vi "initialize_reactors.vi"(8 "ERROR IN":errorcluster, 11 "REACTORS TO USE":u32[](array[numeric])) -> (0 "ERROR OUT":errorcluster, 3 "REACTORS":T1)   [LabVIEW 2013]
uses:
  type_defs/reactors.ctl
  type_defs/reactor.ctl
panel:
  in  "SUMMARY STAT":dbl[](array[numeric])
  in  "TIME STAMPS":dbl[](array[numeric])
  in  "LAST MEASUREMENT":dbl[][](array[numeric])
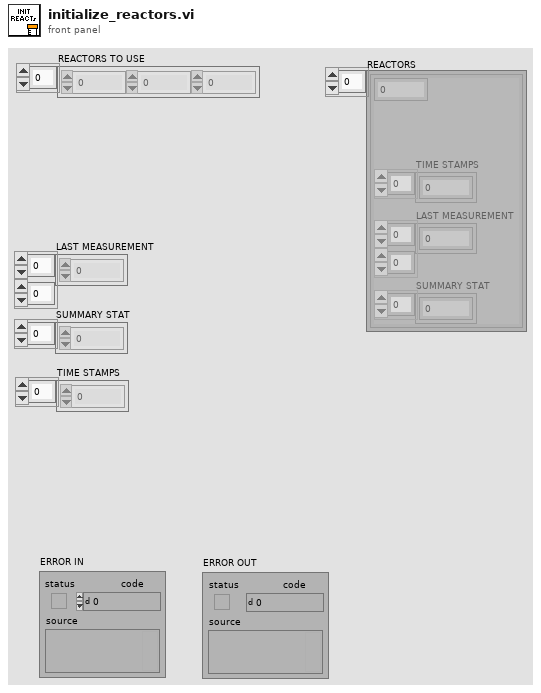
[diagram p1: front panel]
types:
  T1 = typedef "reactors.ctl" = cluster{i32, "TIME STAMPS":dbl[], "LAST MEASUREMENT":T2[][], "SUMMARY STAT":dbl[]}[]
  T2 = typedef "reactor.ctl" = dbl
  T3 = cluster{"Numeric":u32, "TIME STAMPS":dbl[], "LAST MEASUREMENT":dbl[][], "SUMMARY STAT":dbl[]}
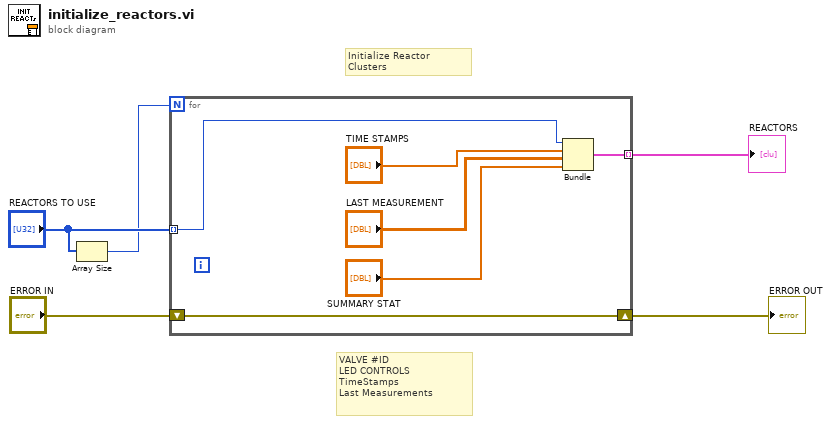
[diagram p0: block diagram]
diagram:
  # "VALVE #ID \nLED CONTROLS\nTimeStamps\nLast Measurements"
  # "Initialize Reactor Clusters"
  n1 = Array Size(array="REACTORS TO USE") -> (size(s)=w2:i32)
  n2 = for {
    N: w2 -> [_]
    tunnel: [w8] -> w1 mode=indexing
    shift-right: [w7] -> w4
    shift-left: "ERROR IN" -> [w7]
    tunnel: "REACTORS TO USE" -> [w6] mode=indexing
    n3 = Bundle("Numeric"=w6, "TIME STAMPS"="TIME STAMPS", "LAST MEASUREMENT"="LAST MEASUREMENT", "SUMMARY STAT"="SUMMARY STAT") -> (w8:T3)  [unwired: 1 in]
  }
  "ERROR OUT" <- w4
  "REACTORS" <- w1
